vi "Network Command Engine.vi"(8 "error in (no error)":errorcluster, 10 "Parameters":T1 {"Config"."Industrial Settings"."Write Refs"."Data Reference" format="%.0x"; "Config"."Industrial Settings"."Read Refs"."Data Reference" format="%.0x"; "Config"."PID Settings"."Read Refs"."Data Reference" format="%.0x"; "Config"."PID Settings"."Write Refs"."Data Reference" format="%.0x"}, 11 "State Variables":T10) -> (0 "error out":errorcluster)   [LabVIEW 2013, in "Control Addon Engine.lvlib"]
uses:
  Control Addon Engine.lvlib
  Inline Async API/Controls/Engine State Variables.ctl
  Stop FG/Stop Global Ref.ctl
  Types/RT Configuration.ctl
  Shared/Types/Gain Schedule.ctl
  Shared/Types/Compiled Settings.ctl
  Shared/Types/Compiled PID Settings.ctl
  <vilib>/NI Veristand/Custom Device API/Block Data Reference.ctl
  <vilib>/NI Veristand/Custom Device API/Data Reference.ctl
  Shared/Types/Compiled Industrial Settings.ctl
  Shared/Types/Compiled Industrial Parameters.ctl
  <vilib>/NI Veristand/Custom Device API/Custom Device Engine Event Ref.ctl
  Stop FG/Stop Global Commands.ctl
  <vilib>/NI Veristand/Custom Device API/Message Response (String).ctl
  Shared/Types/Update Parameters Message.ctl
  Stop FG/Stop FG.lvlib
  Shared/Control Addon Shared.lvlib
  <vilib>/NI Veristand/Custom Device API/Custom Device API.lvlib
  Inline Async API/Inline Async API.lvlib
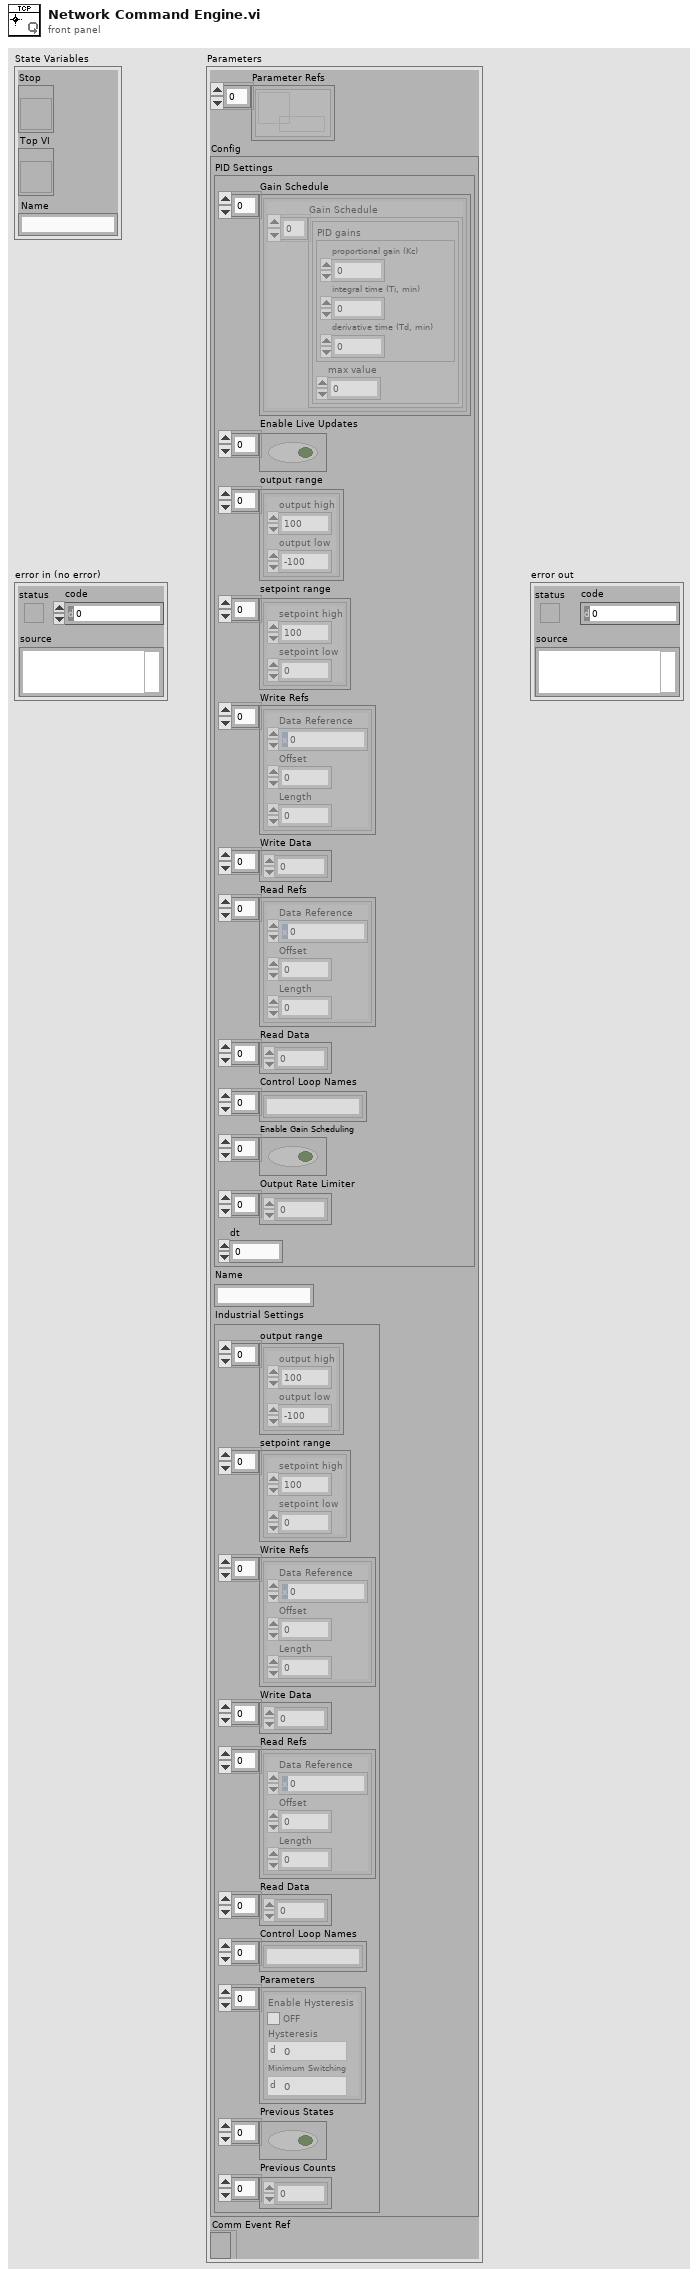
[diagram p1: front panel]
types:
  T1 = typedef "Control Addon Engine.lvlib/RT Configuration.ctl" = cluster{"Parameter Refs":refnum<data-value>[], "Config":T2, "Comm Event Ref":T9}
  T2 = typedef "Control Addon Shared.lvlib/Compiled Settings.ctl" = cluster{"PID Settings":T3, "Name":string, "Industrial Settings":T7}
  T3 = typedef "Control Addon Shared.lvlib/Compiled PID Settings.ctl" = cluster{"Gain Schedule":T4[], "Enable Live Updates":bool[], "output range":cluster{"output high":dbl, "output low":dbl}[], "setpoint range":cluster{"setpoint high":dbl, "setpoint low":dbl}[], "Write Refs":T5[], "Write Data":dbl[], "Read Refs":T5[], "Read Data":dbl[], "Control Loop Names":string[], "Enable Gain Scheduling":bool[], "Output Rate Limiter":dbl[], "dt":dbl}
  T4 = typedef "Control Addon Shared.lvlib/Gain Schedule.ctl" = cluster{"Gain Schedule":cluster{"PID gains":cluster{"proportional gain (Kc)":dbl, "integral time (Ti, min)":dbl, "derivative time (Td, min)":dbl}, "max value":dbl}[]}
  T5 = typedef "Custom Device API.lvlib/Block Data Reference.ctl" = cluster{"Data Reference":T6, "Offset":i32, "Length":i32}
  T6 = typedef "Custom Device API.lvlib/Data Reference.ctl" = i32
  T7 = typedef "Control Addon Shared.lvlib/Compiled Industrial Settings.ctl" = cluster{"output range":cluster{"output high":dbl, "output low":dbl}[], "setpoint range":cluster{"setpoint high":dbl, "setpoint low":dbl}[], "Write Refs":T5[], "Write Data":dbl[], "Read Refs":T5[], "Read Data":dbl[], "Control Loop Names":string[], "Parameters":T8[], "Previous States":bool[], "Previous Counts":u64[]}
  T8 = typedef "Control Addon Shared.lvlib/Compiled Industrial Parameters.ctl" = cluster{"Enable Hysteresis":bool, "Hysteresis":dbl, "Minimum Switching":u64}
  T9 = typedef "Custom Device API.lvlib/Custom Device Engine Event Ref.ctl" = refnum<event-registration>
  T10 = typedef "Control Addon Engine.lvlib/Inline Async API.lvlib/Engine State Variables.ctl" = cluster{"Stop":T11, "Top VI":refnum<vi>, "Name":string}
  T11 = typedef "Control Addon Engine.lvlib/Stop FG.lvlib/Stop Global Ref.ctl" = refnum<vi>
  T12 = typedef "Control Addon Engine.lvlib/Stop FG.lvlib/Stop Global Commands.ctl" = enum16{"Write", "Read", "Reset"}
  T13 = typedef "Custom Device API.lvlib/Message Response (String).ctl" = cluster{"Response":string, "Error":errorcluster}
  T14 = typedef "Control Addon Shared.lvlib/Update Parameters Message.ctl" = cluster{"Control Loop":string, "Gain Schedule":cluster{"PID gains":cluster{"proportional gain (Kc)":dbl, "integral time (Ti, min)":dbl, "derivative time (Td, min)":dbl}, "max value":dbl}[]}
  T15 = typedef "Control Addon Shared.lvlib/Get Settings Message.ctl" = cluster{"Control Loop Names":string[], "Enable Live Updates":bool[], "Gain Schedule":T4[], "Enable Gain Scheduling":bool[]}
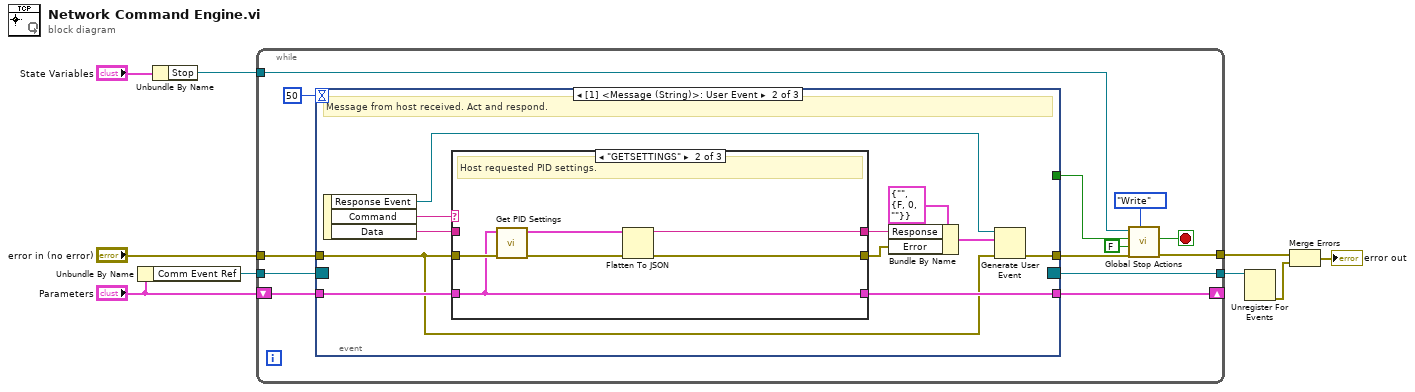
[diagram p0: block diagram]
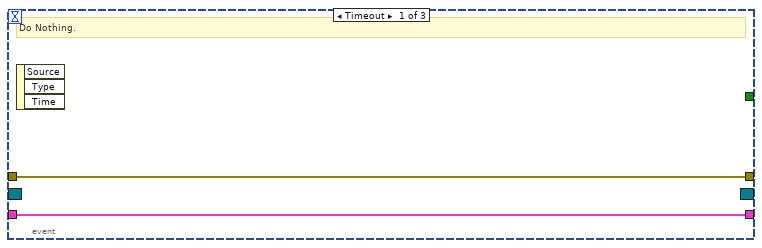
[diagram p2: hidden frame]
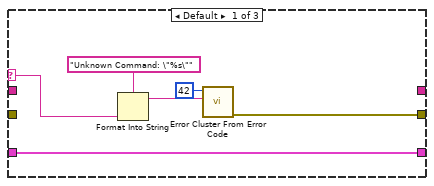
[diagram p3: hidden frame]
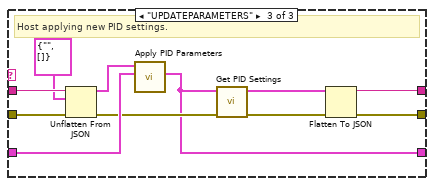
[diagram p4: hidden frame]
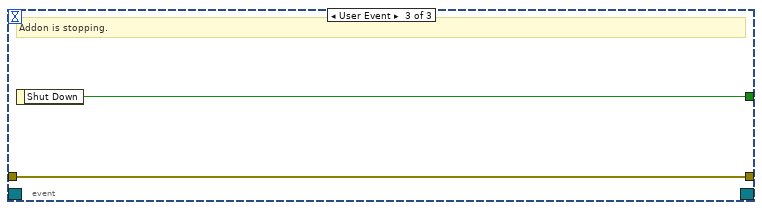
[diagram p5: hidden frame]
diagram:
  n1 = Unbundle By Name("Parameters") -> ("Comm Event Ref"=w5:T9)
  n2 = Unbundle By Name("State Variables") -> ("Stop"=w9:T11)
  n3 = while {
    tunnel: "error in (no error)" -> [w15]
    tunnel: [w18] -> w1
    tunnel: w9 -> [w19]
    shift-right: [w16] -> _
    shift-left: "Parameters" -> [w17]
    tunnel: w5 -> [w13]
    tunnel: [w10] -> w4
    stop <- w20 stop-if-true
    n4 = event shown="[1] <Message (String)>: User Event" {
      selector: w13 -> [_ _ _]
      dyn-events: [_ _ _] -> w10
      timeout: u32 50 ("STM Update Rate") -> [_ _ _]
      tunnel: [w23 w26 w60] -> w21
      tunnel: w17 -> [w24 w35 _]
      tunnel: [w24 w34 _] -> w16
      tunnel: w15 -> [w23 w25 w60]
      tunnel: [_ _ w59] -> w11
      event Timeout {
        # "Do Nothing."
        n5 = event-data() -> ()  [unwired: 1 in, 3 out]
      }
      event User Event {
        # "Message from host received. Act and respond."
        n6 = event-data() -> ("Response Event"=w29:refnum<user-event>, "Command"=w32:string, "Data"=w33:string)  [unwired: 1 in]
        n7 = case shown="\"GETSETTINGS\"" w32 {
          selector: w32 -> [w36 _ _]
          tunnel: w25 -> [_ w47 w52]
          tunnel: [w37 w43 w50] -> w31
          tunnel: w33 -> [_ _ w57]
          tunnel: w35 -> [w41 w46 w58]
          tunnel: [w41 w46 w54] -> w34
          tunnel: [_ w42 w48] -> w30
          frame Default {
            n8 = Format Into String(format string="Unknown Command: \"%s\"", w36) -> (resulting string=w38:string)  [unwired: 2 in, 1 out]
            n9 = call <vilib>:"Error Cluster From Error Code.vi"("error message (\"\")"=w38, "error code (0)"=42) -> ("error out"=w37:errorcluster)  [unwired: 7 in]
          }
          frame "GETSETTINGS" {
            # "Host requested PID settings."
            n10 = call "Get PID Settings.vi"("error in (no error)"=w47, "Parameters"=w46) -> ("error out"=w44:errorcluster, "PID Settings"=w45:T15)  [unwired: 8 in]
            n11 = Flatten To JSON(anything=w45, error in (no error)=w44) -> (JSON string=w42:string, 11:w43:errorcluster)  [unwired: 1 in]
          }
          frame "UPDATEPARAMETERS" {
            # "Host applying new PID settings."
            n12 = Unflatten From JSON(JSON string=w57, type and defaults=T14 {"Control Loop"="", "Gain Schedule"=[]}, error in (no error)=w52) -> (value=w56:T14, error out=w55:errorcluster)  [unwired: 4 in]
            n13 = call "Apply PID Parameters.vi"("Parameters in"=w58, "UpdateParameters"=w56) -> ("Parameters out"=w54:T1)  [unwired: 9 in]
            n14 = call "Get PID Settings.vi"("error in (no error)"=w55, "Parameters"=w54) -> ("error out"=w51:errorcluster, "PID Settings"=w49:T15)  [unwired: 8 in]
            n15 = Flatten To JSON(anything=w49, error in (no error)=w51) -> (JSON string=w48:string, 11:w50:errorcluster)  [unwired: 1 in]
          }
        }
        n16 = Bundle By Name(cluster=T13 {"Response"="", "Error"={"status"=FALSE, "code"=0, "source"=""}} ("event data"), "Response"=w30, "Error"=w31) -> (w27:T13)
        n17 = Generate User Event(user event=w29, event data cluster=w27, error in=w25) -> (error out=w26:errorcluster)  [unwired: 1 in, 1 out]
      }
      event User Event {
        # "Addon is stopping."
        n18 = event-data() -> ("Shut Down"=w59:bool)  [unwired: 1 in]
      }
    }
    n19 = call "Global Stop Actions.vi"("Command"=Stop_Global_Commands."Write", "error in (no error)"=w21, "Stop on Error?"=FALSE, "Stop?"=w11, "vi reference"=w19) -> ("error out"=w18:errorcluster, "Latched Stop"=w20:bool)  [unwired: 4 in, 1 out]
  }
  n20 = Unregister For Events(event registration refnum=w4) -> (error out=w3:errorcluster)  [unwired: 1 in]
  n21 = Merge Errors(w1, w3) -> (→"error out":errorcluster)
